vi "test-discretization.vi"(8 "error in (no error)":errorcluster) -> (0 "error out":errorcluster, 3 "All Tests Passed":bool)   [LabVIEW 2019]
uses:
  <vilib>/Analysis/Matrix/Datatypes/RealMatrix.ctl
  <vilib>/Analysis/baseanly.llb/Real A x B.vi
  <vilib>/Rock Robotics/WPI/ThirdParty/JAS_Junk/TrajLib/MatBuilder_Create.vi
  <vilib>/Rock Robotics/WPI/ThirdParty/JAS_Junk/TrajLib/MatrixHelper_CoerceSize.vi
  <vilib>/Rock Robotics/WPI/ThirdParty/JAS_Junk/TrajLib/Matrix_Exp.vi
  <vilib>/Rock Robotics/WPI/ThirdParty/JAS_Junk/TrajLib/Matrix_AssignBlock.vi
  <vilib>/Rock Robotics/WPI/ThirdParty/JAS_Junk/TrajLib/Matrix_ExtractFrom.vi
  <vilib>/Analysis/7linalg.llb/Transpose Matrix.vi
  <vilib>/Analysis/7linalg.llb/Real Transpose Matrix.vi
  <vilib>/Rock Robotics/WPI/ThirdParty/JAS_Junk/TrajLib/Matrix_Ident.vi
  <vilib>/Analysis/7linalg.llb/Matrix Exp.vi
  <vilib>/Analysis/7linalg.llb/Real Matrix Exp.vi
  <vilib>/Analysis/Matrix/Numeric/Multiply/Multiply.vi
  <vilib>/Analysis/Matrix/Numeric/Multiply/Multiply - RM,R.vi
  <vilib>/Analysis/7linalg.llb/Create Special Matrix.vi
  <vilib>/Analysis/7linalg.llb/Create Special Real Matrix.vi
  <vilib>/Analysis/Matrix/Numeric/Add/Add - RM,RM.vi
  <vilib>/Analysis/Matrix/Comparison/Equal/Equal - RM,RM.vi
  <vilib>/Rock Robotics/WPI/ThirdParty/JAS_Junk/TrajLib/Trajectory_Library.lvlib
  <vilib>/Analysis/NI_AALBase.lvlib
  <vilib>/Analysis/Matrix/NI_Matrix.lvlib
panel:
  out "X1Discrete 11":T1
  out "DiscB  11":T1
  out "Passed 11":bool
  out "DiscA  11":T1
  out "Passed 10":bool
  out "DiscA  10":T1
  out "Passed 16":bool
  out "DiscR  16":T1
  out "A+B Should be":T1
  out "A + B":T1
  out "Test x passed":bool
  out "Test 3 passed":bool
  out "Test Passed 2":bool
  out "Test Passed 1":bool
  out "Test Passed 0":bool
  out "AQ Passed":bool
  out "AQ - DiscQ":T1
  out "AQ - DiscA":T1
  out "AB-Taylor-Passed":bool
  out "ABTaylor-DiscB":T1
  out "ABTaylor - DiscA":T1
  out "AB-passed":bool
  out "AB-DiscB":T1
  out "AB - DiscA":T1
  out "x1-Disc":T1
  out "DiscA Error":bool
  out "DiscA":T1
  out "Cost Mat":T1
  out "CoVar Mat":T1
  # "1.0,   0.0,    0.0\n\n0.0,     4.0,   0.0, ;\n\n0.0,     0.0,  9.0;"
  # "1.0,      0.0,      0.0, \n\n0.0,   1.0 / 4.0,   0.0, \n\n0.0,       0.0,      1.0 / 9.0,"
  # "VecBuilder.fill(\n          x0.get(0, 0) + 1.0 * x0.get(1, 0), \n          x0.get(1, 0));"
  # "2,\n1"
  # "x0.get(0, 0) + x0.get(1, 0) + 0.5 * u.get(0, 0), \n\nx0.get(0, 0) + u.get(0, 0))"
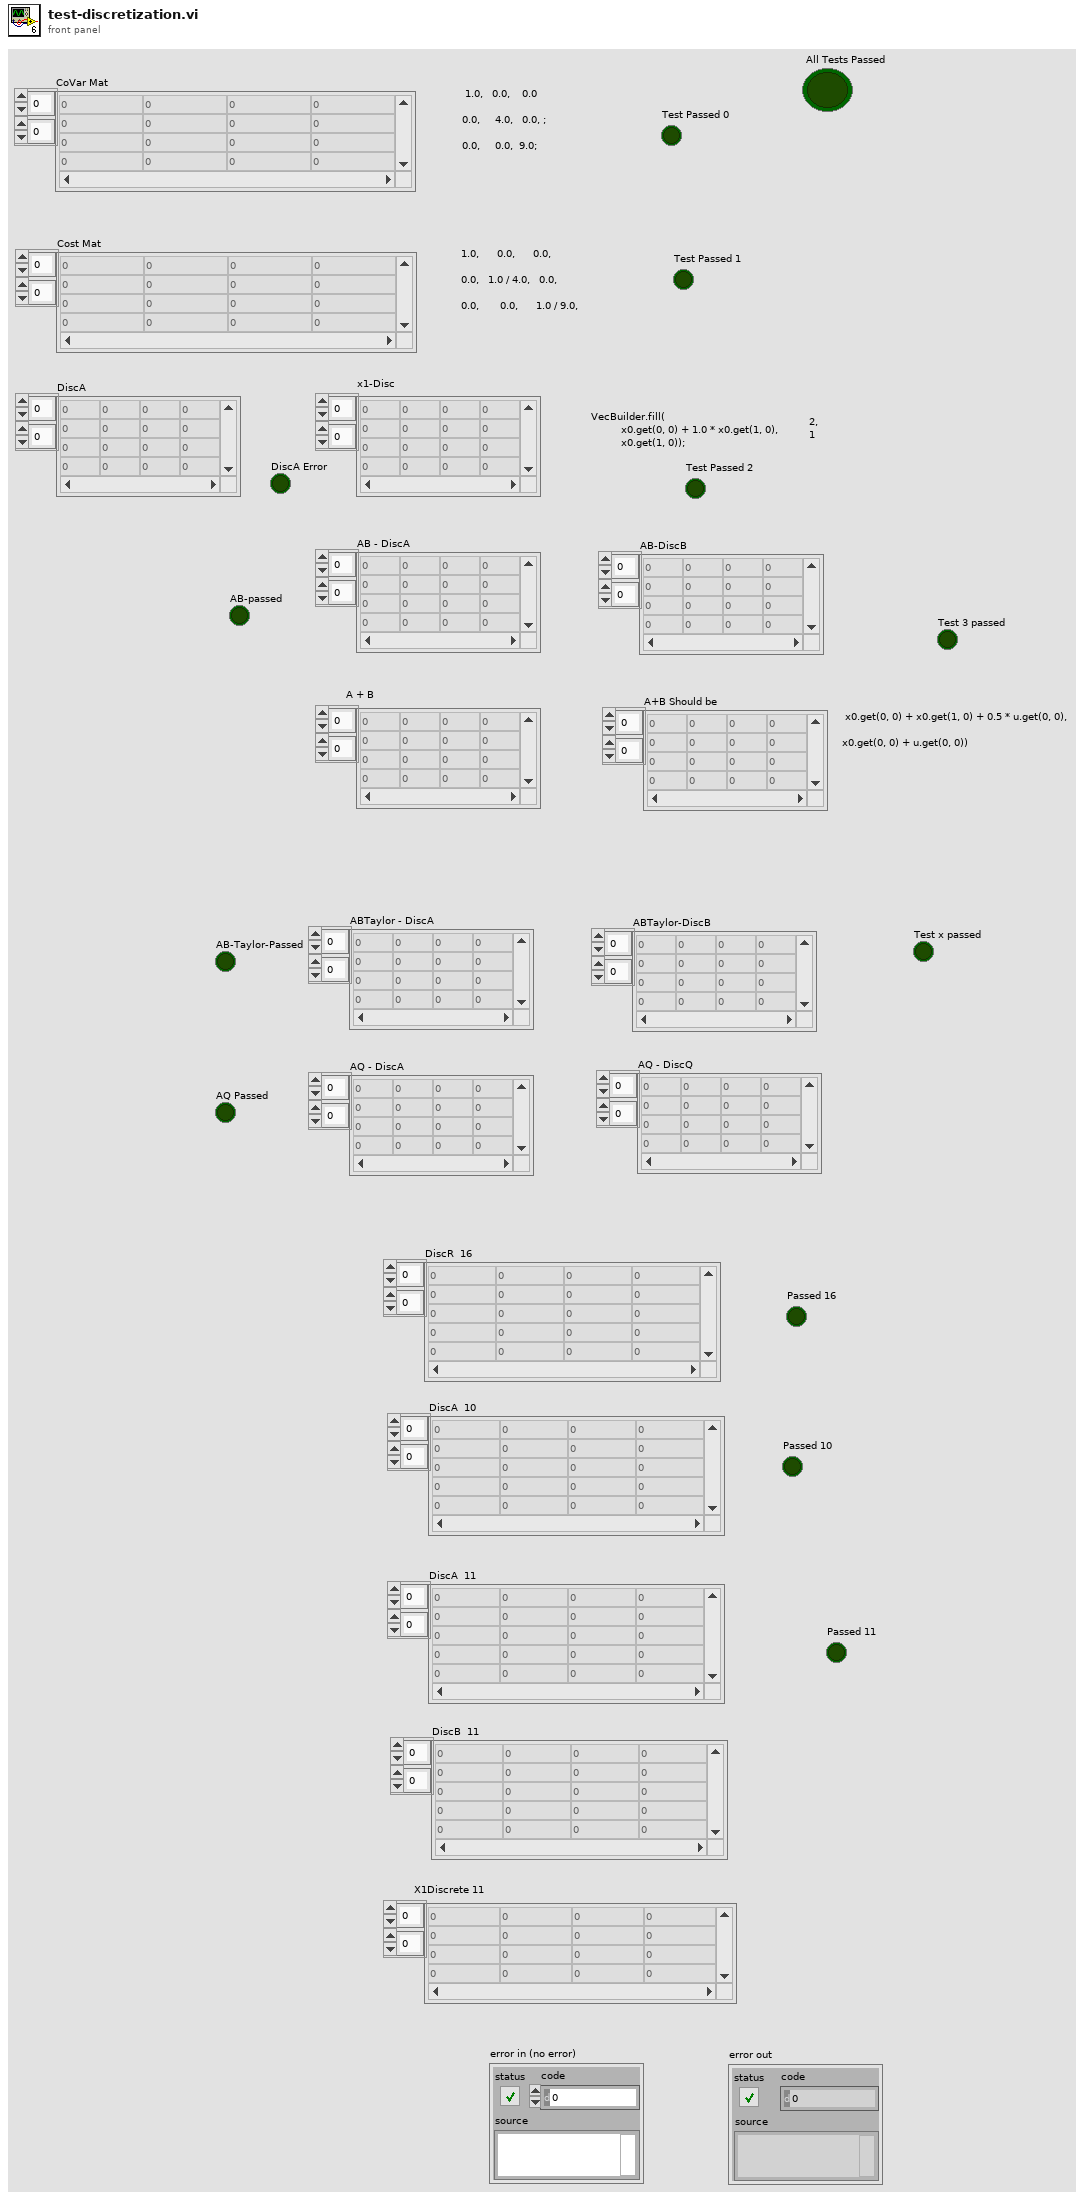
[diagram p1: front panel]
types:
  T1 = typedef "NI_Matrix.lvlib/RealMatrix.ctl" = dbl[][]
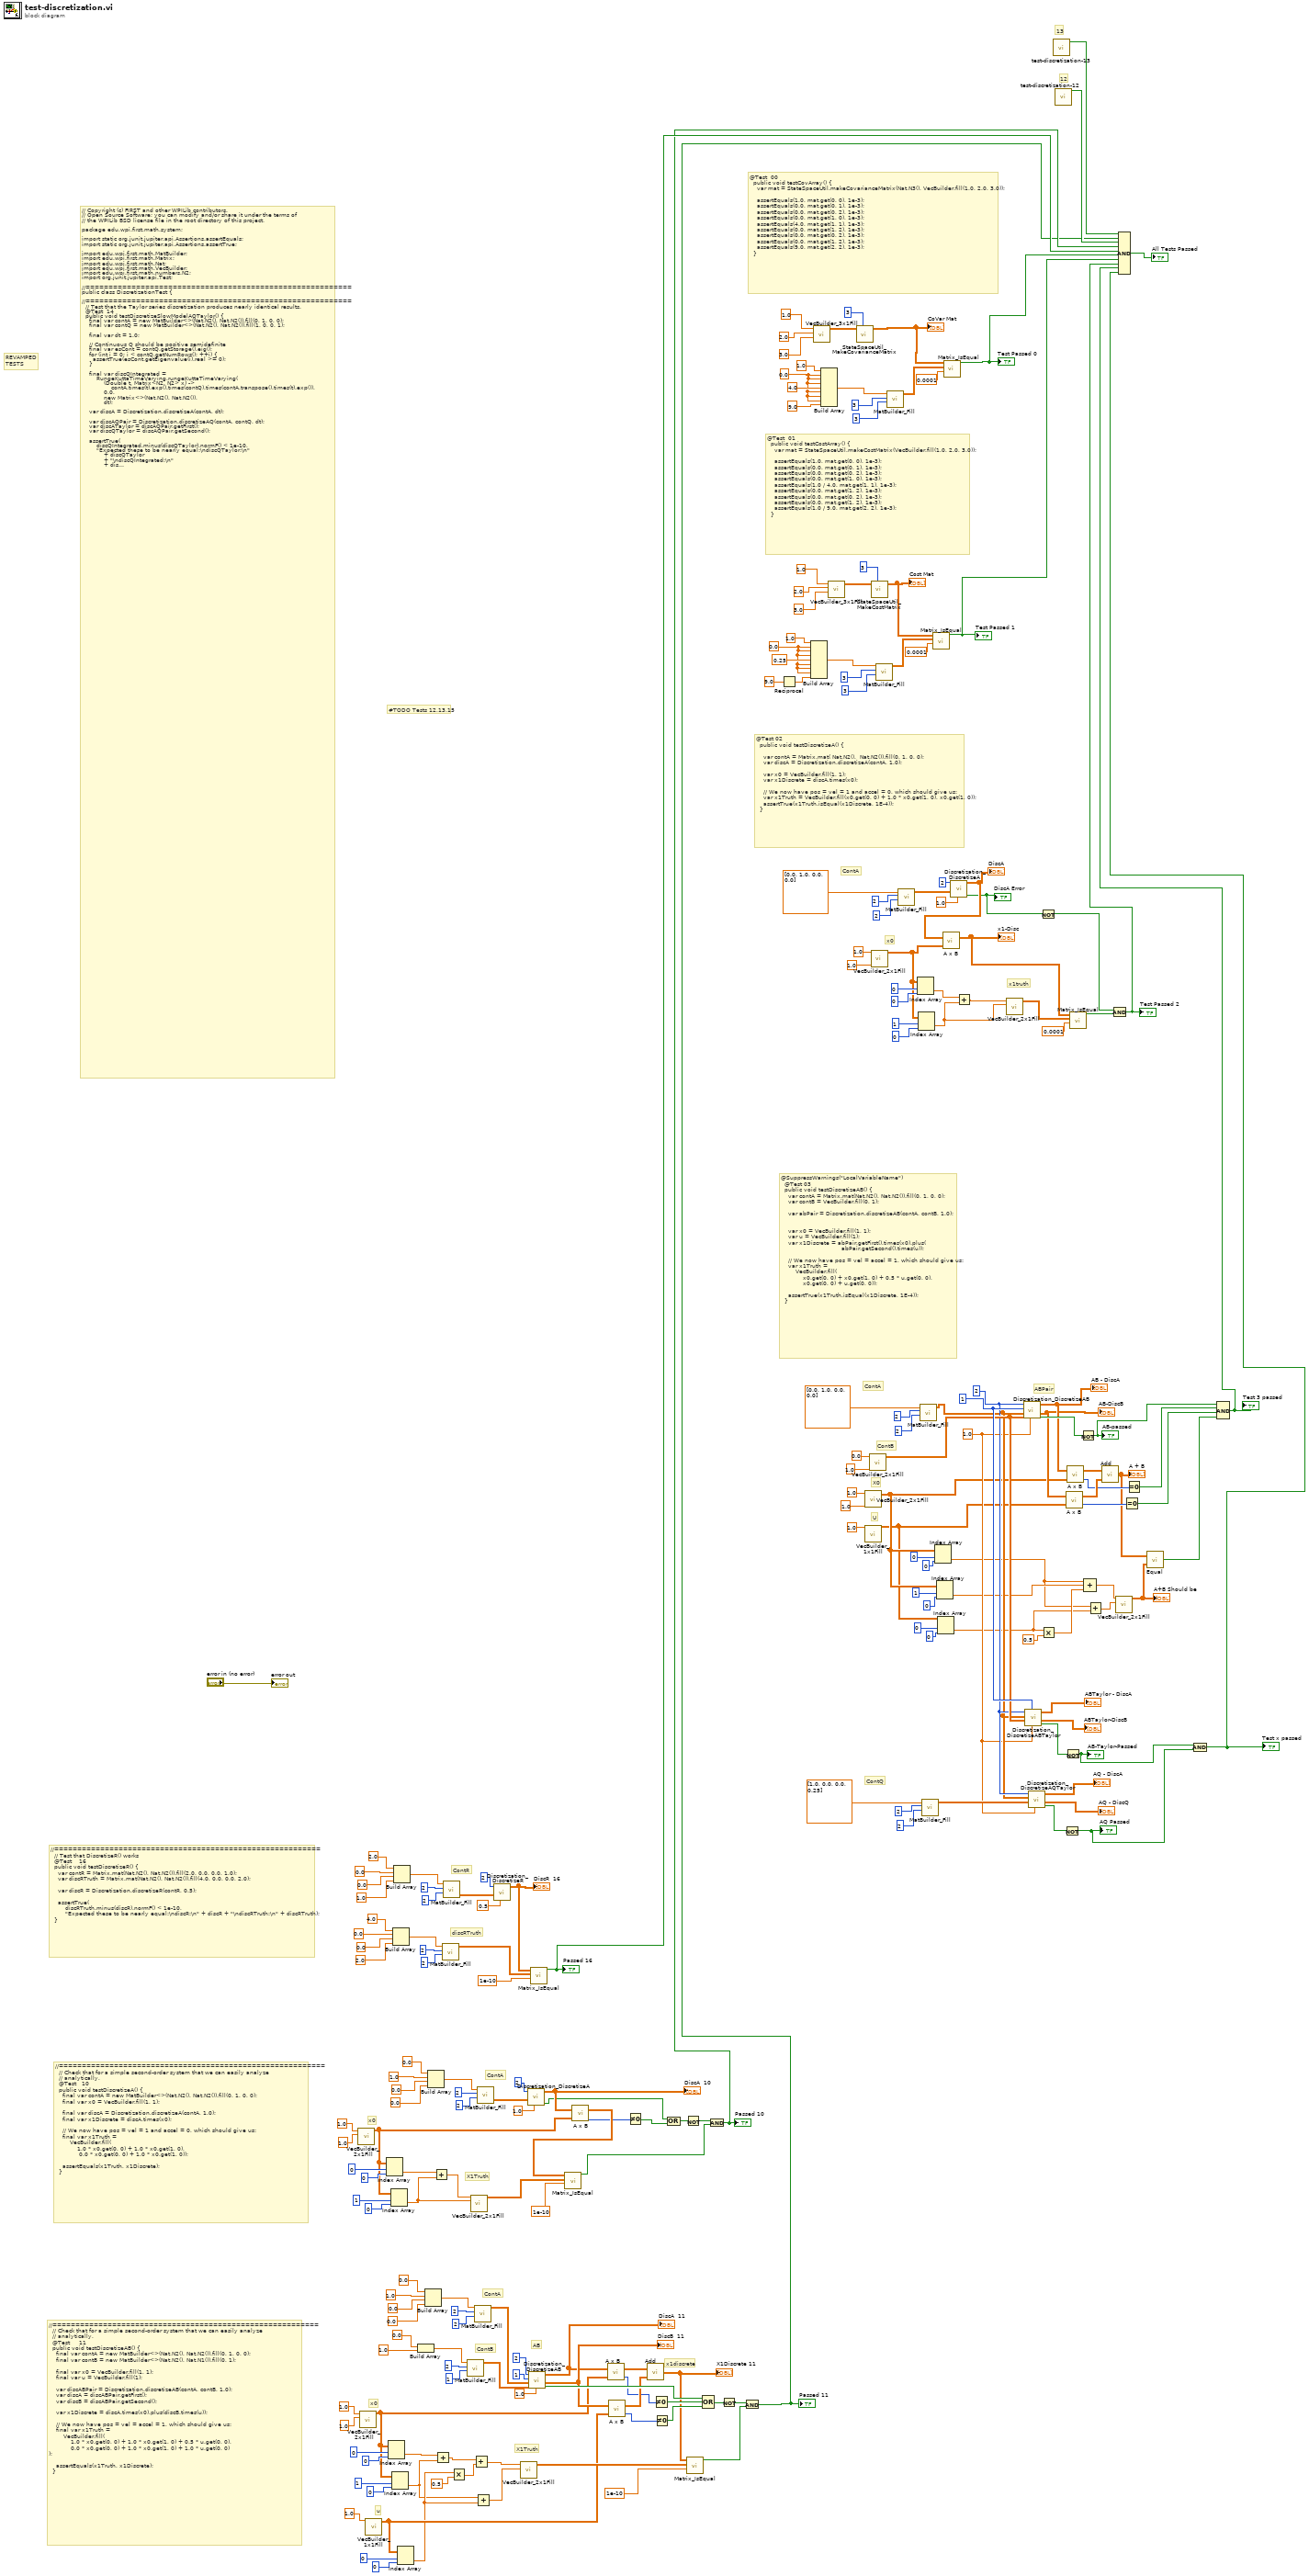
[diagram p0: block diagram]
diagram:
  w168 = 0.0 ("element")
  w178 = 0.0 ("element")
  w186 = 1.0 ("dT_Seconds")
  w196 = 1 ("Inputs")
  w189 = 2 ("States")
  # "13"
  # "#TODO Tests 12,13,15"
  # "AB"
  # "12"
  # "x1discrete"
  # "u"
  # "ContB"
  # "X1Truth"
  # "x0"
  # "ContA"
  # "//==========================================================\n  // Check that for a simple second-order system that we can easily analyze\n  // analytically,\n  @Test     11\n  public void testDiscretizeAB() {\n    final var contA = new MatBuilder<>(Nat.N2(), Nat.N2()).fill(0, 1, 0, 0);\n    final var contB = new MatBuilder<>(Nat.N2(), Nat.N1()).fill(0, 1);\n\n    final var x0 = VecBuilder.fill(1, 1);\n    final var u = VecBuilder.fill(1);\n\n    var discABPair = Discretization.discretizeAB(contA, contB, 1.0);\n    var discA = discABPair.getFirst();\n    var discB = discABPair.getSecond();\n\n    var x1Discrete = discA.times(x0).plus(discB.times(u));\n\n    // We now have pos = vel = accel = 1, which should give us:\n    final var x1Truth =\n        VecBuilder.fill(\n            1.0 * x0.get(0, 0) + 1.0 * x0.get(1, 0) + 0.5 * u.get(0, 0),\n            0.0 * x0.get(0, 0) + 1.0 * x0.get(1, 0) + 1.0 * u.get(0, 0)\n);\n\n    assertEquals(x1Truth, x1Discrete);\n  }"
  # "X1Truth"
  # "x0"
  # "ContA"
  # "//==========================================================\n  // Check that for a simple second-order system that we can easily analyze\n  // analytically,\n  @Test   10\n  public void testDiscretizeA() {\n    final var contA = new MatBuilder<>(Nat.N2(), Nat.N2()).fill(0, 1, 0, 0);\n    final var x0 = VecBuilder.fill(1, 1);\n\n    final var discA = Discretization.discretizeA(contA, 1.0);\n    final var x1Discrete = discA.times(x0);\n\n    // We now have pos = vel = 1 and accel = 0, which should give us:\n    final var x1Truth =\n        VecBuilder.fill(\n            1.0 * x0.get(0, 0) + 1.0 * x0.get(1, 0), \n             0.0 * x0.get(0, 0) + 1.0 * x0.get(1, 0));\n\n    assertEquals(x1Truth, x1Discrete);\n  }"
  # "discRTruth"
  # "ContR"
  # "//==========================================================\n  // Test that DiscretizeR() works\n  @Test    16\n  public void testDiscretizeR() {\n    var contR = Matrix.mat(Nat.N2(), Nat.N2()).fill(2.0, 0.0, 0.0, 1.0);\n    var discRTruth = Matrix.mat(Nat.N2(), Nat.N2()).fill(4.0, 0.0, 0.0, 2.0);\n\n    var discR = Discretization.discretizeR(contR, 0.5);\n\n    assertTrue(\n        discRTruth.minus(discR).normF() < 1e-10,\n        \"Expected these to be nearly equal:\\ndiscR:\\n\" + discR + \"\\ndiscRTruth:\\n\" + discRTruth);\n  }"
  # "REVAMPED\nTESTS"
  # "// Copyright (c) FIRST and other WPILib contributors.\n// Open Source Software; you can modify and/or share it under the terms of\n// the WPILib BSD license file in the root directory of this project.\n\npackage edu.wpi.first.math.system;\n\nimport static org.junit.jupiter.api.Assertions.assertEquals;\nimport static org.junit.jupiter.api.Assertions.assertTrue;\n\nimport edu.wpi.first.math.MatBuilder;\nimport edu.wpi.first.math.Matrix;\nimport edu.wpi.first.math.Nat;\nimport edu.wpi.first.math.VecBuilder;\nimport edu.wpi.first.math.numbers.N2;\nimport org.junit.jupiter.api.Test;\n\n//==========================================================\npublic class DiscretizationTest {\n\n//==========================================================\n  // Test that the Taylor series discretization produces nearly identical results.\n  @Test  14\n  public void testDiscretizeSlowModelAQTaylor() {\n    final var contA = new MatBuilder<>(Nat.N2(), Nat.N2()).fill(0, 1, 0, 0);\n    final var contQ = new MatBuilder<>(Nat.N2(), Nat.N2()).fill(1, 0, 0, 1);\n\n    final var dt = 1.0;\n\n    // Continuous Q should be positive semidefinite\n    final var esCont = contQ.getStorage().eig();\n    for (int i = 0; i < contQ.getNumRows(); ++i) {\n      assertTrue(esCont.getEigenvalue(i).real >= 0);\n    }\n\n    final var discQIntegrated =\n        RungeKuttaTimeVarying.rungeKuttaTimeVarying(\n            (Double t, Matrix<N2, N2> x) ->\n                contA.times(t).exp().times(contQ).times(contA.transpose().times(t).exp()),\n            0.0,\n            new Matrix<>(Nat.N2(), Nat.N2()),\n            dt);\n\n    var discA = Discretization.discretizeA(contA, dt);\n\n    var discAQPair = Discretization.discretizeAQ(contA, contQ, dt);\n    var discATaylor = discAQPair.getFirst();\n    var discQTaylor = discAQPair.getSecond();\n\n    assertTrue(\n        discQIntegrated.minus(discQTaylor).normF() < 1e-10,\n        \"Expected these to be nearly equal:\\ndiscQTaylor:\\n\"\n            + discQTaylor\n            + \"\\ndiscQIntegrated:\\n\"\n            + discQIntegrated);\n    assertTrue(discA.minus(discATaylor).normF() < 1e-10);\n\n    // Discrete Q should be positive semidefinite\n    final var esDisc = discQTaylor.getStorage().eig();\n    for (int i = 0; i < discQTaylor.getNumRows(); ++i) {\n      assertTrue(esDisc.getEigenvalue(i).real >= 0);\n    }\n  }\n\n//==========================================================\n  // Test that the Taylor series discretization produces nearly identical results.\n  @Test  15\n  public void testDiscretizeFastModelAQTaylor() {\n    final var contA = new MatBuilder<>(Nat.N2(), Nat.N2()).fill(0, 1, 0, -1500);\n    final var contQ = new MatBuilder<>(Nat.N2(), Nat.N2()).fill(0.0025, 0, 0, 1);\n\n    final var dt = 0.005;\n\n    // Continuous Q should be positive semidefinite\n    final var esCont = contQ.getStorage().eig();\n    for (int i = 0; i < contQ.getNumRows(); ++i) {\n      assertTrue(esCont.getEigenvalue(i).real >= 0);\n    }\n\n    final var discQIntegrated =\n        RungeKuttaTimeVarying.rungeKuttaTimeVarying(\n            (Double t, Matrix<N2, N2> x) ->\n                contA.times(t).exp().times(contQ).times(contA.transpose().times(t).exp()),\n            0.0,\n            new Matrix<>(Nat.N2(), Nat.N2()),\n            dt);\n\n    var discA = Discretization.discretizeA(contA, dt);\n\n    var discAQPair = Discretization.discretizeAQ(contA, contQ, dt);\n    var discATaylor = discAQPair.getFirst();\n    var discQTaylor = discAQPair.getSecond();\n\n    assertTrue(\n        discQIntegrated.minus(discQTaylor).normF() < 1e-3,\n        \"Expected these to be nearly equal:\\ndiscQTaylor:\\n\"\n            + discQTaylor\n            + \"\\ndiscQIntegrated:\\n\"\n            + discQIntegrated);\n    assertTrue(discA.minus(discATaylor).normF() < 1e-10);\n\n    // Discrete Q should be positive semidefinite\n    final var esDisc = discQTaylor.getStorage().eig();\n    for (int i = 0; i < discQTaylor.getNumRows(); ++i) {\n      assertTrue(esDisc.getEigenvalue(i).real >= 0);\n    }\n  }\n\n}"
  # "U"
  # "X0"
  # "ContB"
  # "ABPair"
  # "x1truth"
  # "x0"
  # "ContQ"
  # "ContA"
  # "@SuppressWarnings(\"LocalVariableName\")\n  @Test 03\n  public void testDiscretizeAB() {\n    var contA = Matrix.mat(Nat.N2(), Nat.N2()).fill(0, 1, 0, 0);\n    var contB = VecBuilder.fill(0, 1);\n\n    var abPair = Discretization.discretizeAB(contA, contB, 1.0);\n\n\n    var x0 = VecBuilder.fill(1, 1);\n    var u = VecBuilder.fill(1);\n    var x1Discrete = abPair.getFirst().times(x0).plus(\n                                 abPair.getSecond().times(u));\n\n    // We now have pos = vel = accel = 1, which should give us:\n    var x1Truth =\n        VecBuilder.fill(\n            x0.get(0, 0) + x0.get(1, 0) + 0.5 * u.get(0, 0), \n            x0.get(0, 0) + u.get(0, 0));\n\n    assertTrue(x1Truth.isEqual(x1Discrete, 1E-4));\n  }"
  # "ContA"
  # "@Test 02\n  public void testDiscretizeA() {\n\n    var contA = Matrix.mat( Nat.N2(),  Nat.N2()).fill(0, 1, 0, 0);\n    var discA = Discretization.discretizeA(contA, 1.0);\n\n    var x0 = VecBuilder.fill(1, 1);\n    var x1Discrete = discA.times(x0);\n\n    // We now have pos = vel = 1 and accel = 0, which should give us:\n    var x1Truth = VecBuilder.fill(x0.get(0, 0) + 1.0 * x0.get(1, 0), x0.get(1, 0));\n    assertTrue(x1Truth.isEqual(x1Discrete, 1E-4));\n  }"
  # "@Test  01\n  public void testCostArray() {\n    var mat = StateSpaceUtil.makeCostMatrix(VecBuilder.fill(1.0, 2.0, 3.0));\n\n    assertEquals(1.0, mat.get(0, 0), 1e-3);\n    assertEquals(0.0, mat.get(0, 1), 1e-3);\n    assertEquals(0.0, mat.get(0, 2), 1e-3);\n    assertEquals(0.0, mat.get(1, 0), 1e-3);\n    assertEquals(1.0 / 4.0, mat.get(1, 1), 1e-3);\n    assertEquals(0.0, mat.get(1, 2), 1e-3);\n    assertEquals(0.0, mat.get(0, 2), 1e-3);\n    assertEquals(0.0, mat.get(1, 2), 1e-3);\n    assertEquals(1.0 / 9.0, mat.get(2, 2), 1e-3);\n  }"
  # "@Test  00\n  public void testCovArray() {\n    var mat = StateSpaceUtil.makeCovarianceMatrix(Nat.N3(), VecBuilder.fill(1.0, 2.0, 3.0));\n\n    assertEquals(1.0, mat.get(0, 0), 1e-3);\n    assertEquals(0.0, mat.get(0, 1), 1e-3);\n    assertEquals(0.0, mat.get(0, 2), 1e-3);\n    assertEquals(0.0, mat.get(1, 0), 1e-3);\n    assertEquals(4.0, mat.get(1, 1), 1e-3);\n    assertEquals(0.0, mat.get(1, 2), 1e-3);\n    assertEquals(0.0, mat.get(0, 2), 1e-3);\n    assertEquals(0.0, mat.get(1, 2), 1e-3);\n    assertEquals(9.0, mat.get(2, 2), 1e-3);\n  }"
  n1 = call <vilib>:"VecBuilder_2x1Fill.vi"("R1"=1.0, "R0"=1.0) -> ("output matrix"=w68:T1)  [unwired: 9 in]
  n2 = call <vilib>:"VecBuilder_2x1Fill.vi"("R1"=1.0, "R0"=1.0) -> ("output matrix"=w22:T1)  [unwired: 9 in]
  n3 = call <vilib>:"VecBuilder_1x1Fill.vi"("R0_C0"=1.0 ("R0")) -> ("output matrix"=w13:T1)  [unwired: 10 in]
  n4 = Index Array(array=w68, index (row)=0, index (col)=0) -> (element=w65:dbl)
  n5 = Index Array(array=w22, index (row)=0, index (col)=0) -> (element=w39:dbl)
  n6 = Index Array(array=w68, index (row)=1, index (col)=0) -> (element=w64:dbl)
  n7 = Index Array(array=w22, index (row)=1, index (col)=0) -> (element=w7:dbl)
  n8 = Build Array(4.0 ("element"), 0.0 ("element"), 0.0 ("element"), 2.0 ("element")) -> (w100:dbl[])
  n9 = Build Array(2.0 ("element"), 0.0 ("element"), 0.0 ("element"), 1.0 ("element")) -> (w107:dbl[])
  n10 = Index Array(array=w13, index (row)=0, index (col)=0) -> (element=w8:dbl)
  n11 = Build Array(0.0 ("element"), 1.0 ("element")) -> (w33:dbl[])
  n12 = Build Array(0.0 ("element"), 1.0 ("element"), 0.0 ("element"), 0.0 ("element")) -> (w56:dbl[])
  n13 = Build Array(0.0 ("element"), 1.0 ("element"), 0.0 ("element"), 0.0 ("element")) -> (w86:dbl[])
  n14 = Add(x=w65, y=w64) -> (x+y=w66:dbl)
  n15 = Add(x=w39, y=w7) -> (x+y=w10:dbl)
  n16 = call <vilib>:"MatBuilder_Fill.vi"("Columns"=2, "Rows"=2, "Value List"=w100) -> ("output matrix"=w89:T1)  [unwired: 8 in]
  n17 = call <vilib>:"MatBuilder_Fill.vi"("Columns"=2, "Rows"=2, "Value List"=w107) -> ("output matrix"=w92:T1)  [unwired: 8 in]
  n18 = Multiply(x=w8, y=0.5) -> (x*y=w11:dbl)
  n19 = call <vilib>:"MatBuilder_Fill.vi"("Columns"=1, "Rows"=2, "Value List"=w33) -> ("output matrix"=w27:T1)  [unwired: 8 in]
  n20 = call <vilib>:"VecBuilder_2x1Fill.vi"("R1"=w64, "R0"=w66) -> ("output matrix"=w67:T1)  [unwired: 9 in]
  n21 = Add(x=w10, y=w11) -> (x+y=w9:dbl)
  n22 = call <vilib>:"MatBuilder_Fill.vi"("Columns"=2, "Rows"=2, "Value List"=w56) -> ("output matrix"=w28:T1)  [unwired: 8 in]
  n23 = Add(x=w7, y=w8) -> (x+y=w6:dbl)
  n24 = call <vilib>:"MatBuilder_Fill.vi"("Columns"=2, "Rows"=2, "Value List"=w86) -> ("output matrix"=w78:T1)  [unwired: 8 in]
  n25 = call <vilib>:"Discretization_DiscretizeR.vi"("dT_Seconds"=0.5, "ContR"=w92, "Outputs"=2) -> ("DiscR"=w91:T1)  [unwired: 7 in, 1 out]
  "DiscR  16" <- w91
  n26 = call <vilib>:"VecBuilder_2x1Fill.vi"("R1"=w6, "R0"=w9) -> ("output matrix"=w40:T1)  [unwired: 9 in]
  n27 = call <vilib>:"Discretization_DiscretizeA.vi"("dT_Seconds"=1.0, "ContA"=w78, "States"=2 ("Outputs")) -> ("Error"=w61:bool, "DiscA"=w73:T1)  [unwired: 7 in]
  "DiscA  10" <- w73
  n28 = call <vilib>:"Discretization_DiscretizeAB.vi"("dT_Seconds"=1.0, "ContB"=w27, "ContA"=w28, "Inputs"=1, "States"=2 ("Outputs")) -> ("Error"=w38:bool, "DiscB"=w24:T1, "DiscA"=w23:T1)  [unwired: 4 in]
  "DiscA  11" <- w23
  "DiscB  11" <- w24
  n29 = call <vilib>:"Matrix_IsEqual.vi"("Tolerance"=1e-10, "other"=w89, "input matrix"=w91) -> ("Equal"=w87:bool)  [unwired: 8 in]
  "Passed 16" <- w87
  n30 = call-poly <vilib>:"A x B.vi"("B"=w68, "A"=w73) -> ("error"=w62:i32, "A x B"=w63:T1)
  n31 = call <vilib>:"Matrix_IsEqual.vi"("Tolerance"=1e-10, "other"=w67, "input matrix"=w63) -> ("Equal"=w57:bool)  [unwired: 8 in]
  n32 = call-poly <vilib>:"A x B.vi"("B"=w22, "A"=w23) -> ("error"=w18:i32, "A x B"=w21:T1)
  n33 = call-poly <vilib>:"A x B.vi"("B"=w13, "A"=w24) -> ("error"=w17:i32, "A x B"=w20:T1)
  n34 = Not Equal To 0?(x=w62) -> (x != 0?=w60:bool)
  n35 = call-poly <vilib>:"Add.vi"("Real Matrix B"=w20, "Real Matrix A"=w21) -> ("A + B"=w16:T1)
  "X1Discrete 11" <- w16
  n36 = Not Equal To 0?(x=w18) -> (x != 0?=w37:bool)
  n37 = Not Equal To 0?(x=w17) -> (x != 0?=w19:bool)
  n38 = Compound Arithmetic op=OR(w61, w60) -> (w59:bool)
  n39 = Not(x=w59) -> (.not. x?=w58:bool)
  n40 = call <vilib>:"Matrix_IsEqual.vi"("Tolerance"=1e-10, "other"=w40, "input matrix"=w16) -> ("Equal"=w34:bool)  [unwired: 8 in]
  n41 = Compound Arithmetic op=OR(w38, w37, w19) -> (w36:bool)
  n42 = And(x=w58, y=w57) -> (x .and. y?=w5:bool)
  "Passed 10" <- w5
  n43 = Not(x=w36) -> (.not. x?=w35:bool)
  n44 = And(x=w35, y=w34) -> (x .and. y?=w2:bool)
  "Passed 11" <- w2
  n45 = Reciprocal(x=9.0 ("element")) -> (1/x=w164:dbl)
  n46 = Build Array(1.0 ("element"), w168, w168, w168, 0.25 ("element"), w168, w168, w168, w164) -> (w171:dbl[])
  n47 = call <vilib>:"VecBuilder_3x1Fill.vi"("R2"=3.0, "R1"=2.0, "R0"=1.0) -> ("output matrix"=w217:T1)  [unwired: 8 in]
  n48 = Build Array(1.0 ("element"), w178, w178, w178, 4.0 ("element"), w178, w178, w178, 9.0 ("element")) -> (w181:dbl[])
  n49 = call <vilib>:"VecBuilder_3x1Fill.vi"("R2"=3.0, "R1"=2.0, "R0"=1.0) -> ("output matrix"=w212:T1)  [unwired: 8 in]
  n50 = call <vilib>:"StateSpaceUtil_MakeCovarianceMatrix.vi"("States"=3, "StdDevs"=w217) -> ("Covariance Matrix"=w176:T1)  [unwired: 8 in, 1 out]
  "CoVar Mat" <- w176
  n51 = call <vilib>:"VecBuilder_2x1Fill.vi"("R1"=1.0, "R0"=1.0 ("R0_C0")) -> ("output matrix"=w119:T1)  [unwired: 9 in]
  n52 = call <vilib>:"VecBuilder_1x1Fill.vi"("R0_C0"=1.0) -> ("output matrix"=w118:T1)  [unwired: 10 in]
  n53 = call <vilib>:"VecBuilder_2x1Fill.vi"("R1"=1.0, "R0"=0.0 ("R0_C0")) -> ("output matrix"=w195:T1)  [unwired: 9 in]
  n54 = call <vilib>:"StateSpaceUtil_MakeCostMatrix.vi"("States"=3, "Costs"=w212) -> ("Costs Matrix"=w163:T1)  [unwired: 8 in, 1 out]
  "Cost Mat" <- w163
  n55 = call <vilib>:"VecBuilder_2x1Fill.vi"("R1"=1.0, "R0"=1.0 ("R0_C0")) -> ("output matrix"=w157:T1)  [unwired: 9 in]
  n56 = call <vilib>:"MatBuilder_Fill.vi"("Columns"=3, "Rows"=3, "Value List"=w171) -> ("output matrix"=w167:T1)  [unwired: 8 in]
  n57 = call <vilib>:"MatBuilder_Fill.vi"("Columns"=3, "Rows"=3, "Value List"=w181) -> ("output matrix"=w175:T1)  [unwired: 8 in]
  n58 = call <vilib>:"MatBuilder_Fill.vi"("Columns"=2, "Rows"=2, "Value List"=dbl[] [0.0, 1.0, 0.0, 0.0]) -> ("output matrix"=w205:T1)  [unwired: 8 in]
  n59 = Index Array(array=w157, index (row)=0, index (col)=0) -> (element=w156:dbl)
  n60 = Index Array(array=w157, index (row)=1, index (col)=0) -> (element=w154:dbl)
  n61 = call <vilib>:"MatBuilder_Fill.vi"("Columns"=2, "Rows"=2, "Value List"=dbl[] [0.0, 1.0, 0.0, 0.0]) -> ("output matrix"=w188:T1)  [unwired: 8 in]
  n62 = call <vilib>:"MatBuilder_Fill.vi"("Columns"=2, "Rows"=2, "Value List"=dbl[] [1.0, 0.0, 0.0, 0.25]) -> ("output matrix"=w187:T1)  [unwired: 8 in]
  n63 = call <vilib>:"Matrix_IsEqual.vi"("Tolerance"=0.0001, "other"=w167, "input matrix"=w163) -> ("Equal"=w147:bool)  [unwired: 8 in]
  "Test Passed 1" <- w147
  n64 = Index Array(array=w119, index (row)=0, index (col)=0) -> (element=w112:dbl)
  n65 = Index Array(array=w119, index (row)=1, index (col)=0) -> (element=w116:dbl)
  n66 = Index Array(array=w118, index (row)=0, index (col)=0) -> (element=w111:dbl)
  n67 = call <vilib>:"Matrix_IsEqual.vi"("Tolerance"=0.0001, "other"=w175, "input matrix"=w176) -> ("Equal"=w148:bool)  [unwired: 8 in]
  "Test Passed 0" <- w148
  n68 = call <vilib>:"Discretization_DiscretizeA.vi"("dT_Seconds"=1.0, "ContA"=w205, "States"=2) -> ("Error"=w150:bool, "DiscA"=w202:T1)  [unwired: 7 in]
  "DiscA" <- w202
  "DiscA Error" <- w150
  n69 = call-poly <vilib>:"A x B.vi"("B"=w157, "A"=w202) -> ("A x B"=w153:T1)  [unwired: 1 out]
  "x1-Disc" <- w153
  n70 = Add(x=w156, y=w154) -> (x+y=w155:dbl)
  n71 = call <vilib>:"VecBuilder_2x1Fill.vi"("R1"=w154, "R0"=w155) -> ("output matrix"=w152:T1)  [unwired: 9 in]
  n72 = call <vilib>:"Discretization_DiscretizeAB.vi"("dT_Seconds"=w186, "ContB"=w195, "ContA"=w188, "Inputs"=w196, "States"=w189) -> ("Error"=w144:bool, "DiscB"=w134:T1, "DiscA"=w138:T1)  [unwired: 4 in]
  "AB - DiscA" <- w138
  "AB-DiscB" <- w134
  n73 = call <vilib>:"Discretization_DiscretizeABTaylor.vi"("dT_Seconds"=w186, "Inputs"=w196, "ContB"=w195, "ContA"=w188, "States"=w189) -> ("Error"=w143:bool, "DiscB"=→"ABTaylor-DiscB":T1, "DiscA"=→"ABTaylor - DiscA":T1)  [unwired: 4 in]
  n74 = call <vilib>:"Discretization_DiscretizeAQTaylor.vi"("dT_Seconds"=w186, "ContQ"=w187, "ContA"=w188, "States"=w189) -> ("Error"=w141:bool, "DiscQ"=→"AQ - DiscQ":T1, "DiscA"=→"AQ - DiscA":T1)  [unwired: 5 in]
  n75 = Not(x=w150) -> (.not. x?=w149:bool)
  n76 = Multiply(x=w111, y=0.5) -> (x*y=w115:dbl)
  n77 = call "test-discretization-13.vi"() -> ("All Tests Passed"=w1:bool)  [unwired: 10 in, 1 out]
  n78 = call "test-discretization-12.vi"() -> ("All Tests Passed"=w3:bool)  [unwired: 10 in, 1 out]
  n79 = Not(x=w141) -> (.not. x?=w139:bool)
  "AQ Passed" <- w139
  n80 = Not(x=w143) -> (.not. x?=w140:bool)
  "AB-Taylor-Passed" <- w140
  n81 = call-poly <vilib>:"A x B.vi"("B"=w118, "A"=w134) -> ("error"=w130:i32, "A x B"=w132:T1)
  n82 = call-poly <vilib>:"A x B.vi"("B"=w119, "A"=w138) -> ("error"=w131:i32, "A x B"=w133:T1)
  n83 = call <vilib>:"Matrix_IsEqual.vi"("Tolerance"=0.0001, "other"=w152, "input matrix"=w153) -> ("Equal"=w151:bool)  [unwired: 8 in]
  n84 = Not(x=w144) -> (.not. x?=w142:bool)
  "AB-passed" <- w142
  n85 = Compound Arithmetic op=ADD(w112, w116, w115) -> (w114:dbl)
  n86 = Add(x=w112, y=w111) -> (x+y=w113:dbl)
  n87 = call-poly <vilib>:"Add.vi"("Real Matrix B"=w132, "Real Matrix A"=w133) -> ("A + B"=w109:T1)
  "A + B" <- w109
  n88 = Compound Arithmetic op=AND(w149, w151) -> (w146:bool)
  "Test Passed 2" <- w146
  n89 = call <vilib>:"VecBuilder_2x1Fill.vi"("R1"=w113, "R0"=w114) -> ("output matrix"=w110:T1)  [unwired: 9 in]
  "A+B Should be" <- w110
  n90 = Equal To 0?(x=w130) -> (x = 0?=w128:bool)
  n91 = Equal To 0?(x=w131) -> (x = 0?=w129:bool)
  n92 = call-poly <vilib>:"Equal.vi"("Real Matrix B"=w110, "Real Matrix A"=w109) -> ("A = B?"=w108:bool)
  n93 = Compound Arithmetic op=AND(w140, w139) -> (w126:bool)
  "Test x passed" <- w126
  n94 = Compound Arithmetic op=AND(w142, w129, w128, w108) -> (w127:bool)
  "Test 3 passed" <- w127
  n95 = Compound Arithmetic op=AND(w1, w2, w3, w5, w87, w148, w147, w146, w127, w126) -> (→"All Tests Passed":bool)
  "error out" <- "error in (no error)"
